vi "Get MSS.vi"(8 "error in (no error)":errorcluster, 11 "Study Base in":refnum<class "Study Base.lvclass">) -> (0 "error out":errorcluster, 2 "HAL GOOP4.lvlib:Measure and Stimulus Subsystems":refnum<class "Measure and Stimulus Subsystems.lvclass">, 3 "Study Base out":refnum<class "Study Base.lvclass">)   [LabVIEW 2023, in "HAL GOOP4.lvlib" / "Study Base.lvclass"]
uses:
  Study Base.lvclass
  Study Base.lvclass/Study Base.ctl
  Measure and Stimulus Subsystems/Measure and Stimulus Subsystems.lvclass
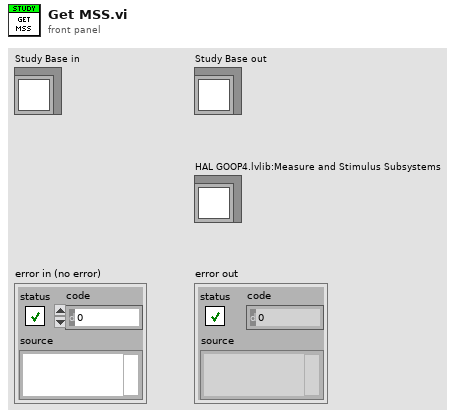
[diagram p1: front panel]
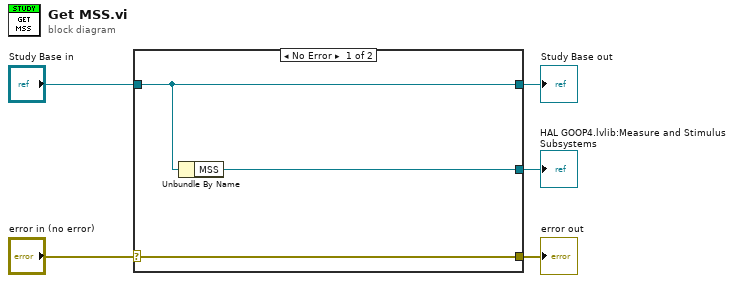
[diagram p0: block diagram]
diagram:
  n1 = case shown="No Error" "error in (no error)" {
    selector: "error in (no error)" -> [w8 w9]
    tunnel: [w8 w9] -> w4
    tunnel: [w7 w10] -> w2
    tunnel: "Study Base in" -> [w7 w10]
    tunnel: [w6 _] -> w1
    frame No Error {
      n2 = Unbundle By Name(w7) -> ("MSS"=w6:refnum<class "Measure and Stimulus Subsystems.lvclass">)
    }
    frame Error {
    }
  }
  "error out" <- w4
  "Study Base out" <- w2
  "HAL GOOP4.lvlib:Measure and Stimulus Subsystems" <- w1
